vi "Label_Prefix.vi"() -> (0 "Label Prefix String":string)   [LabVIEW 2016, in "Hardware.lvlib" / "Displacement Sensor.lvlib" / "DispSnsr Configuration.lvclass"]
uses:
  <userlib>/Common Components/Hardware/Displacement Sensor/DispSnsr Config/DispSnsr Configuration.lvclass
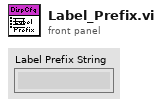
[diagram p1: front panel]
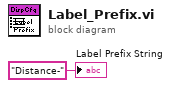
[diagram p0: block diagram]
diagram:
  "Label Prefix String" <- "Distance-" ("Label Prefix String")
